vi "Stop Core.vi"(10 "final error code":i32, 11 "Panel Manager Controller in":refnum<class "Panel Manager Controller.lvclass">) -> (3 "Panel Manager Controller out":refnum<class "Panel Manager Controller.lvclass">)   [LabVIEW 2015, in "Panel Manager Controller.lvclass"]
doc: "(<B>Filename</B>: Actor Framework.lvlib:Actor.lvclass:Stop Core.vi)\n\nDefines what the actor does before it stops. Use the <B>final error code</B> input to determine whether the actor shut down in response to an error.\n\nBy default, this method does nothing. A descendant class may override it to define behavior, such as shutting down any processes the actor initiated in its override of the Actor Core method."
uses:
  Panel Manager Controller.lvclass
  Panel Manager Controller.lvclass/Panel Manager Controller.ctl
  <vilib>/ActorFramework/Stop Msg/Stop Msg.lvclass/Stop Msg.ctl
  <vilib>/ActorFramework/Message Enqueuer/Message Enqueuer.lvclass/Message Enqueuer.ctl
  <vilib>/ActorFramework/Message Enqueuer/Enqueue Critical.vi
  <vilib>/ActorFramework/Message Priority Queue/Priority Enqueue.vi
  <vilib>/ActorFramework/Actor/Actor.lvclass
  <vilib>/ActorFramework/Stop Msg/Stop Msg.lvclass
  _Depences/Panel API/Panel Control_Interface/Panel_interface/Panel Controller Interface.lvclass
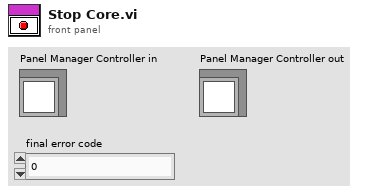
[diagram p1: front panel]
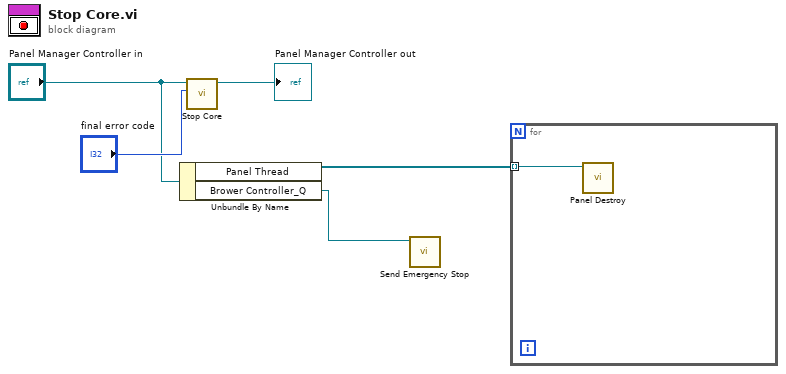
[diagram p0: block diagram]
diagram:
  n1 = Unbundle By Name("Panel Manager Controller in") -> ("Panel Thread"=w2:refnum<class "Panel Controller Interface.lvclass">[], "Brower Controller_Q"=w1:refnum<class "Message Enqueuer.lvclass">)
  n2 = call-parent "Stop Core.vi"("final error code"="final error code", "Actor in"="Panel Manager Controller in") -> ("Actor out"=→"Panel Manager Controller out":refnum<class "Panel Manager Controller.lvclass">)  [unwired: 9 in]
  n3 = call <vilib>:"Send Emergency Stop.vi"("Message Enqueuer"=w1) -> ()  [unwired: 10 in, 1 out]
  n4 = for {
    tunnel: w2 -> [w6] mode=indexing
    n5 = call-dynamic "Panel Destroy.vi"("Panel in"=w6) -> ()  [unwired: 9 in, 2 out]
  }
